vi "Get Turret Filter.vi"(0 "Notifier Name In":string, 11 "Error In":errorcluster) -> (4 "Notifier Name Out":string, 8 "Turret Filter Index":u8, 15 "Error Out":errorcluster)   [LabVIEW 2020]
uses:
  Microscopes Type Defs/Microscope Notifier.ctl
  Microscopes Type Defs/Microscope Actions.ctl
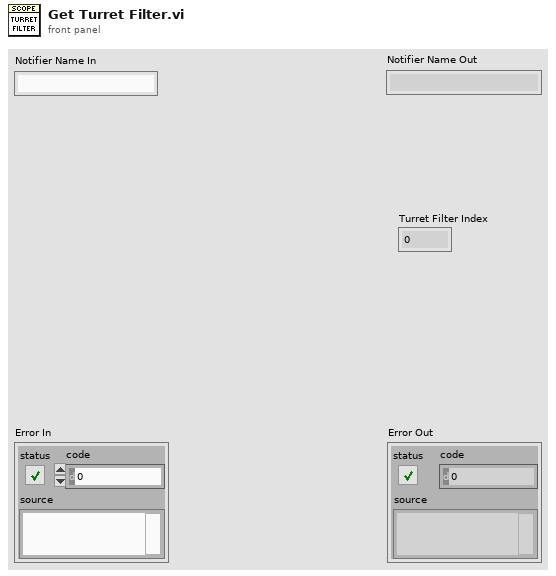
[diagram p1: front panel]
types:
  T1 = typedef "Microscope Notifier.ctl" = cluster{"Actions":T2, "Action Done":bool, "Objective Index":u8, "Objective Z Position (um)":dbl, "Lamp Index":u8, "Lamp State":bool, "Output Port":u8, "Shutter Index":u8, "Shutter State":bool, "Dichroic Wheel Position":u8, "Parameter":string, "Parameter Value":string, "Base Locked?":bool, "Obj Speed":u32, "Obj Acceleration":u32, "Obj Deceleration":u32, "Lamp Power (%)":dbl, "Dichroic Wheel Index":u8}
  T2 = typedef "Microscope Actions.ctl" = enum16{"Do Nothing", "Lock Base", "Lock Focus Knob", "Get Objective Index", "Get Objective Z Position", "Get Lamp State", "Get Lamp Power", "Get Output Port", "Get Shutter State", "Get Dichroic Wheel Position", "Set Lamp Index", "Set Shutter Index", "Set Objective Z Position", "Set Lamp State", "Set Lamp Power", "Set Output Port", "Set Shutter State", "Set Dichroic Wheel Position", "Set Objective", "Abort Move", "Set Parameter", "Get Parameter", "Quit"}
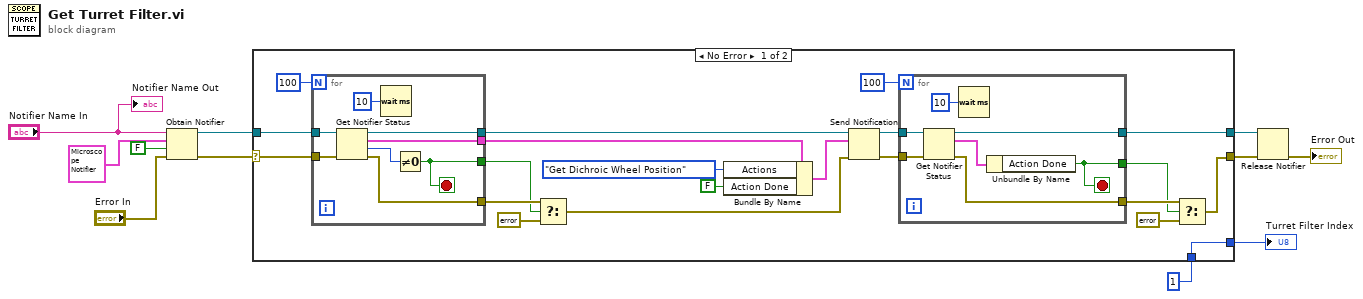
[diagram p0: block diagram]
diagram:
  n1 = Obtain Notifier(name (unnamed)="Notifier Name In", notification data type=T1 {"Actions"=enum."Get Objective Index", "Action Done"=FALSE, "Objective Index"=0, "Objective Z Position (um)"=0.0, "Lamp Index"=0, "Lamp State"=FALSE, "Output Port"=0, "Shutter Index"=0, "Shutter State"=FALSE, "Dichroic Wheel Position"=0, "Parameter"="", "Parameter Value"="", "Base Locked?"=FALSE, "Obj Speed"=0, "Obj Acceleration"=0, "Obj Deceleration"=0, "Lamp Power (%)"=0.0, "Dichroic Wheel Index"=0} ("Microscope Notifier"), create if not found? (T)=FALSE, error in (no error)="Error In") -> (notifier out=w8:refnum<notifier>, error out=w9:errorcluster)  [unwired: 1 out]
  n2 = case shown="No Error" w9 {
    selector: w9 -> [w30 w50]
    tunnel: w8 -> [w32 w49]
    tunnel: [w21 w50] -> w4
    tunnel: [w22 w49] -> w5
    tunnel: u8 1 -> [w17 w48]
    tunnel: [w17 w48] -> w1
    frame No Error {
      n3 = for {
        N: 100 -> [_]
        tunnel: w32 -> [w47]
        tunnel: [w45] -> w18
        tunnel: [w43] -> w28
        tunnel: w30 -> [w42]
        tunnel: [w41] -> w19
        tunnel: [w40] -> w29
        stop <- w45 stop-if-true
        n4 = Get Notifier Status(notifier=w47, error in (no error)=w42) -> (notifier out=w43:refnum<notifier>, current notification=w40:T1, # waiting=w46:i32, error out=w41:errorcluster)  [unwired: 1 out]
        n5 = Wait (ms)(milliseconds to wait=u32 10) -> ()  [unwired: 1 out]
        n6 = Not Equal To 0?(x=w46) -> (x != 0?=w45:bool)
      }
      n7 = Select(t=w19, s=w18, f=errorcluster {"status"=TRUE, "code"=0, "source"="IX81 Base Error: Base busy time out."}) -> (s? t:f=w12:errorcluster)
      n8 = Bundle By Name(cluster=w29, "Actions"=Microscope_Actions."Get Dichroic Wheel Position", "Action Done"=FALSE) -> (w27:T1)
      n9 = Send Notification(notification=w27, notifier=w28, error in (no error)=w12) -> (notifier out=w23:refnum<notifier>, error out=w26:errorcluster)
      n10 = for {
        N: 100 -> [_]
        tunnel: w23 -> [w39]
        tunnel: [w37] -> w22
        tunnel: w26 -> [w36]
        tunnel: [w35] -> w15
        tunnel: [w33] -> w14
        stop <- w33 stop-if-true
        n11 = Get Notifier Status(notifier=w39, error in (no error)=w36) -> (notifier out=w37:refnum<notifier>, current notification=w34:T1, error out=w35:errorcluster)  [unwired: 2 out]
        n12 = Wait (ms)(milliseconds to wait=u32 10) -> ()  [unwired: 1 out]
        n13 = Unbundle By Name(w34) -> ("Action Done"=w33:bool)
      }
      n14 = Select(t=w15, s=w14, f=errorcluster {"status"=TRUE, "code"=0, "source"="IX81 Base Error: Action didn't complete."}) -> (s? t:f=w21:errorcluster)
    }
    frame Error {
    }
  }
  "Turret Filter Index" <- w1
  n15 = Release Notifier(notifier=w5, error in (no error)=w4) -> (error out=→"Error Out":errorcluster)  [unwired: 1 in, 2 out]
  "Notifier Name Out" <- "Notifier Name In"
